vi "加B索引.vi"(1 "索引值":u8[](array[numeric])) -> (0 "加B索引值":u8[](array[numeric]))   [LabVIEW 2013]
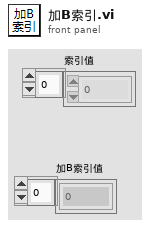
[diagram p1: front panel]
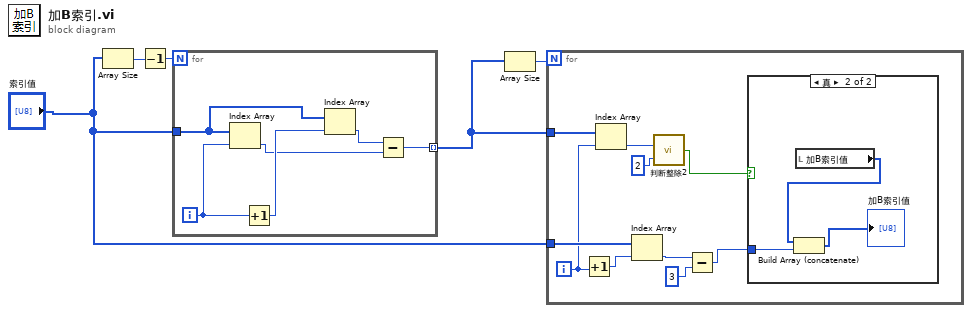
[diagram p0: block diagram]
diagram:
  n1 = Array Size(array="索引值") -> (size(s)=w4:i32)
  n2 = Decrement(x=w4) -> (x-1=w5:i32)
  n3 = for {
    N: w5 -> [_]
    tunnel: "索引值" -> [w11]
    tunnel: [w7] -> w2 mode=indexing
    i -> [w6]
    n4 = Index Array(array=w11, index=w6) -> (element=w8:u8)
    n5 = Increment(x=w6) -> (x+1=w10:i32)
    n6 = Index Array(array=w11, index=w10) -> (element=w9:u8)
    n7 = Subtract(x=w9, y=w8) -> (x-y=w7:u8)
  }
  n8 = Array Size(array=w2) -> (size(s)=w3:i32)
  n9 = for {
    N: w3 -> [_]
    tunnel: w2 -> [w21]
    tunnel: "索引值" -> [w20]
    i -> [w19]
    n10 = Increment(x=w19) -> (x+1=w18:i32)
    n11 = Index Array(array=w21, index=w19) -> (element=w15:u8)
    n12 = Index Array(array=w20, index=w18) -> (element=w17:u8)
    n13 = call "判断整除2.vi"("被除数"=2, "除数"=w15) -> ("布尔 2"=w13:bool)
    n14 = Subtract(x=w17, y=3) -> (x-y=w12:i32)
    n15 = case shown="真" w13 {
      tunnel: w12 -> [_ w24]
      frame False {
      }
      frame True {
        n16 = local read "加B索引值"() -> (w22:u8[])
        n17 = Build Array (concatenate)(w22, w24) -> (→"加B索引值":i32[])
      }
    }
  }
